vi "SwerveModeToDash.vi"(10 "Update?":bool, 11 "SwerveModeIn":T1=enum."Home") -> (3 "SwerveModeOut":T1=enum."Home")   [LabVIEW 2018]
uses:
  SwerveRotationCalibrate.ctl
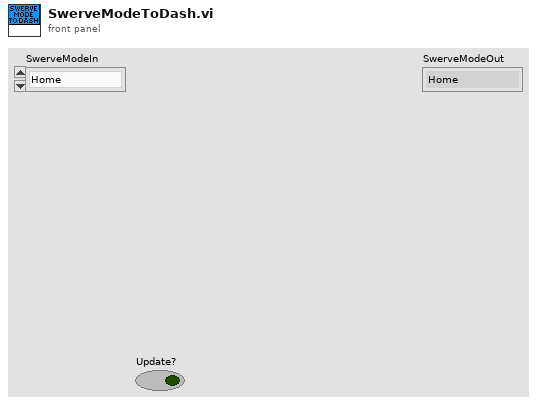
[diagram p1: front panel]
types:
  T1 = typedef "SwerveRotationCalibrate.ctl" = enum16{"Calibrate", "Home", "ManualHome", "ResetQuad", "Drive"}
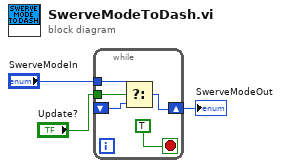
[diagram p0: block diagram]
diagram:
  n1 = while {
    tunnel: "Update?" -> [w8]
    shift-right: [w7] -> w1
    shift-left: _ -> [w6]
    tunnel: "SwerveModeIn" -> [w4]
    stop <- TRUE stop-if-true
    n2 = Select(t=w4, s=w8, f=w6) -> (s? t:f=w7:T1)
  }
  "SwerveModeOut" <- w1
